vi "Get Primary Destination Path.vi"(8 "error in (no error)":errorcluster, 11 "NI_AB_API_SDIST.lvclass in":refnum<class "NI_AB_API_DSDIST.lvclass">) -> (0 "error out":errorcluster, 2 "Primary destination path":path, 3 "NI_AB_API_SDIST.lvclass out":refnum<class "NI_AB_API_DSDIST.lvclass">)   [LabVIEW 2020, in "NI_AB_API_DSDIST.lvclass"]
uses:
  <vilib>/AppBuilder/AB_API/DSDIST/NI_AB_API_DSDIST.lvclass
  <vilib>/AppBuilder/AB_API/SDIST/NI_AB_API_SDIST.lvclass
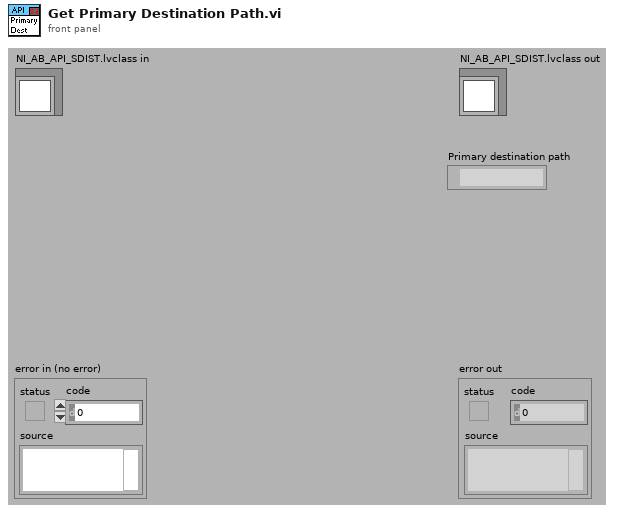
[diagram p1: front panel]
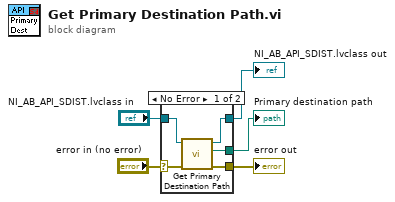
[diagram p0: block diagram]
diagram:
  n1 = case shown="No Error" "error in (no error)" {
    selector: "error in (no error)" -> [w8 w11]
    tunnel: [w7 w11] -> w4
    tunnel: [w9 w12] -> w2
    tunnel: "NI_AB_API_SDIST.lvclass in" -> [w10 w12]
    tunnel: [w6 _] -> w1
    frame No Error {
      n2 = call-parent "Get Primary Destination Path.vi"("error in (no error)"=w8, "NI_AB_API_SDIST in"=w10) -> ("error out"=w7:errorcluster, "Primary destination path"=w6:path, "NI_AB_API_SDIST out"=w9:refnum<class "NI_AB_API_DSDIST.lvclass">)  [unwired: 7 in]
    }
    frame Error {
    }
  }
  "error out" <- w4
  "NI_AB_API_SDIST.lvclass out" <- w2
  "Primary destination path" <- w1
